vi "PauseUIUpdates.vi"(8 "error in (no error)":errorcluster, 11 "Calendar in":refnum<class "Calendar.lvclass">) -> (0 "error out":errorcluster, 3 "Calendar out":refnum<class "Calendar.lvclass">)   [LabVIEW 2020, in "Calendar.lvclass"]
uses:
  Calendar.lvclass
  C:/Program Files/National Instruments/LabVIEW 2020/vi.lib/QSI/QControls/QControl Classes/Generic/Generic.lvclass
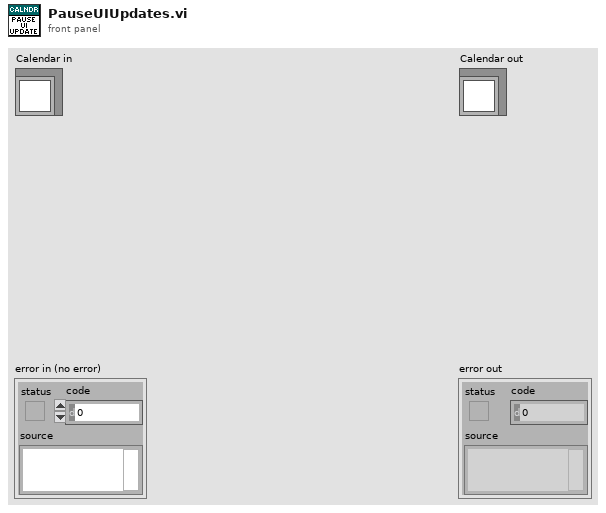
[diagram p1: front panel]
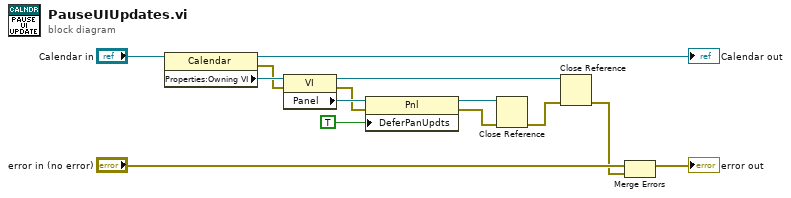
[diagram p0: block diagram]
diagram:
  n1 = property class="Calendar"(reference="Calendar in") -> (reference out=→"Calendar out":refnum<class "Calendar.lvclass">, error out=w11:errorcluster, "Properties:Owning VI"=w12:refnum<vi>)  [unwired: 1 in]
  n2 = property class="VI"(reference=w12, error in=w11) -> (reference out=w5:refnum<vi>, error out=w9:errorcluster, "Panel"=w10:refnum<vi>)
  n3 = property class="Pnl"(reference=w10, error in=w9, "DeferPanUpdts"=TRUE ("Defer Panel Updates")) -> (reference out=w7:refnum<vi>, error out=w6:errorcluster)
  n4 = Close Reference(reference=w7, error in (no error)=w6) -> (error out=w4:errorcluster)
  n5 = Close Reference(reference=w5, error in (no error)=w4) -> (error out=w2:errorcluster)
  n6 = Merge Errors("error in (no error)", w2) -> (→"error out":errorcluster)
